vi "System Messages.vi"(5 "Source Name":string, 7 "Source Type":T1, 8 "error in (no error)":errorcluster, 9 "Payload":variant, 10 "Identifier":string) -> (0 "error out":errorcluster)   [LabVIEW 2020, in "TCP Sever.lvlib"]
doc: "_____\nCreated using Delacor QMH Event Scripter 5.0.0.112."
uses:
  TCP Sever.lvlib
  Libraries/hse-libraries/hse-dqmh/Controls/System Message Source.ctl
  System Messages Argument--cluster.ctl
  Libraries/hse-libraries/hse-dqmh/hse-dqmh.lvlib
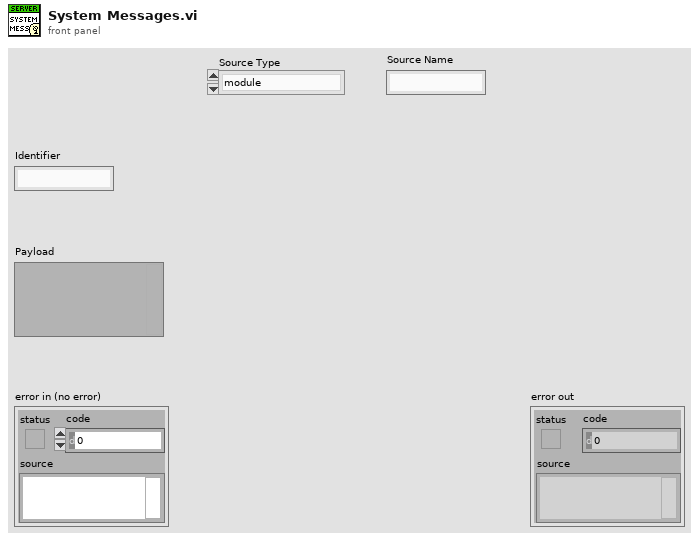
[diagram p1: front panel]
types:
  T1 = typedef "hse-dqmh.lvlib/System Message Source.ctl" = enum16{"module", "application", "network"}
  T2 = typedef "TCP Sever.lvlib/System Messages Argument--cluster.ctl" = cluster{"Identifier":string, "Payload":variant, "Source Type":T1, "Source Name":string}
  T3 = typedef "TCP Sever.lvlib/Broadcast Events--cluster.ctl" = cluster{"Module Did Init":refnum<user-event>, "Status Updated":refnum<user-event>, "Error Reported":refnum<user-event>, "Did Something":refnum<user-event>, "Module Did Stop":refnum<user-event>, "Update Module Execution Status":refnum<user-event>, "System Messages":refnum<user-event>}
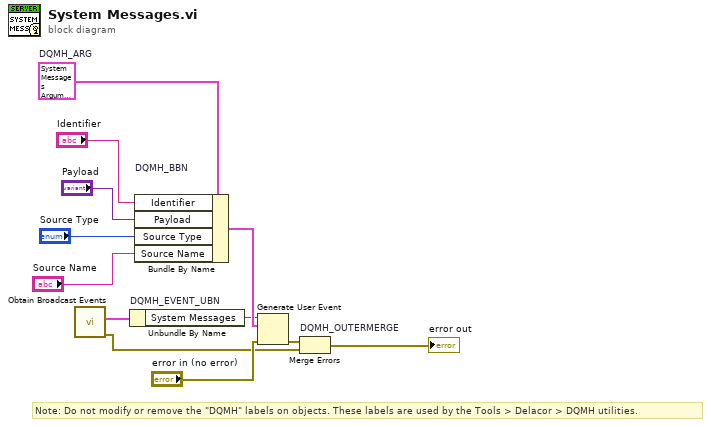
[diagram p0: block diagram]
diagram:
  w7 = T2 {"Identifier"="", "Payload"=variant, "Source Type"=enum."module", "Source Name"=""}  # DQMH_ARG
  # "Note: Do not modify or remove the \"DQMH\" labels on objects. These labels are used by the Tools > Delacor > DQMH utilities."
  n1 = call "Obtain Broadcast Events.vi"() -> ("error out"=w2:errorcluster, "TCP Sever Broadcast Events"=w1:T3)  [unwired: 10 in]
  n2 = Unbundle By Name "DQMH_EVENT_UBN"(w1) -> ("System Messages"=w9:refnum<user-event>)
  n3 = Bundle By Name "DQMH_BBN"(cluster=w7, "Identifier"="Identifier", "Payload"="Payload", "Source Type"="Source Type", "Source Name"="Source Name") -> (w10:T2)
  n4 = Generate User Event(user event=w9, event data cluster=w10, error in="error in (no error)") -> (error out=w8:errorcluster)  [unwired: 1 in, 1 out]
  n5 = Merge Errors "DQMH_OUTERMERGE"(w8, w2) -> (→"error out":errorcluster)
